vi "plot y axis pixel widths.vi"(9 "Scale.Bounds:Area Width":u32, 11 "Axis.Visible":bool) -> (3 "title width":i32)   [LabVIEW 2021, in "RocketPlot.lvlib"]
uses:
  RocketPlot.lvlib
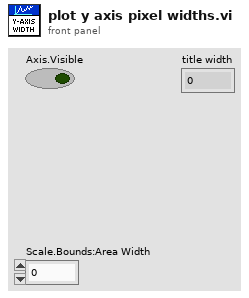
[diagram p1: front panel]
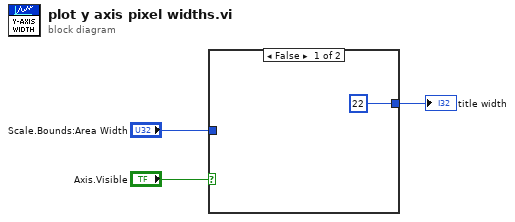
[diagram p0: block diagram]
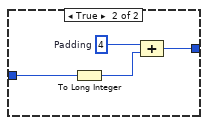
[diagram p2: hidden frame]
diagram:
  n1 = case shown="False" "Axis.Visible" {
    tunnel: [22 w7] -> w2
    tunnel: "Scale.Bounds:Area Width" -> [_ w6]
    frame False {
    }
    frame True {
      w8 = 4  # Padding
      n2 = To Long Integer(number=w6) -> (32bit integer=w5:i32)
      n3 = Compound Arithmetic op=ADD(w8, w5) -> (w7:i32)
    }
  }
  "title width" <- w2
